vi "DSP_SetSamplesPerRecordAdj.vi"(2 "error in (no error)":errorcluster, 3 "value":u32, 4 "Board Handle":u64) -> (0 "error out":errorcluster, 1 "Board Handle Out":u64)   [LabVIEW 2009]
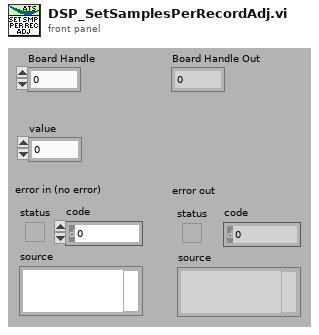
[diagram p1: front panel]
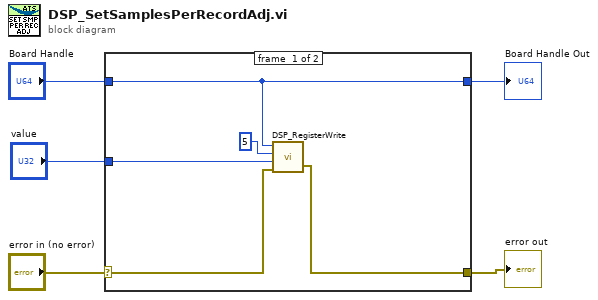
[diagram p0: block diagram]
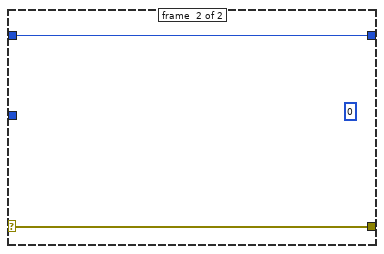
[diagram p2: hidden frame]
diagram:
  n1 = case shown="No Error" "error in (no error)" {
    selector: "error in (no error)" -> [w10 w12]
    tunnel: [w9 w12] -> w4
    tunnel: [w8 w11] -> w3
    tunnel: "Board Handle" -> [w8 w11]
    tunnel: "value" -> [w6 _]
    frame #0 {
      n2 = call "DSP_RegisterWrite.vi"("error in (no error)"=w10, "Value"=w6, "Offset"=u32 5, "Board Handle"=w8) -> ("error out"=w9:errorcluster)  [unwired: 1 out]
    }
    frame #1 {
      (unwired) u32 0
    }
  }
  "Board Handle Out" <- w3
  "error out" <- w4
